vi "Radau5_Choose Step Size.vi"(0 "step size":dbl, 1 "Step index":i32, 2 "Index of Y":i8[](array[numeric]), 5 "old step size":dbl, 7 "ErrorTolerance":dbl[](array[numeric]), 9 "Local error":dbl[](array[numeric]), 11 "Old Local error":dbl[](array[numeric])) -> (4 "New step size":dbl)   [LabVIEW 2017, in "NI_DAE.lvlib"]
uses:
  <vilib>/gmath/NI_DAE.lvlib
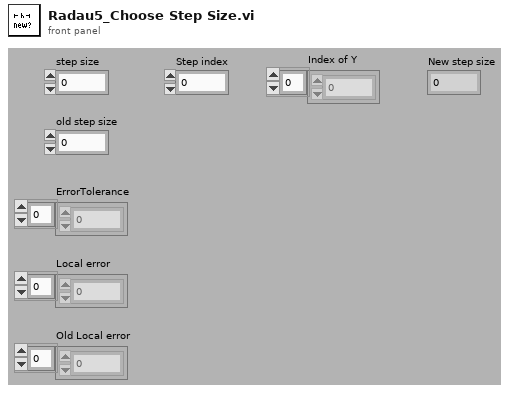
[diagram p1: front panel]
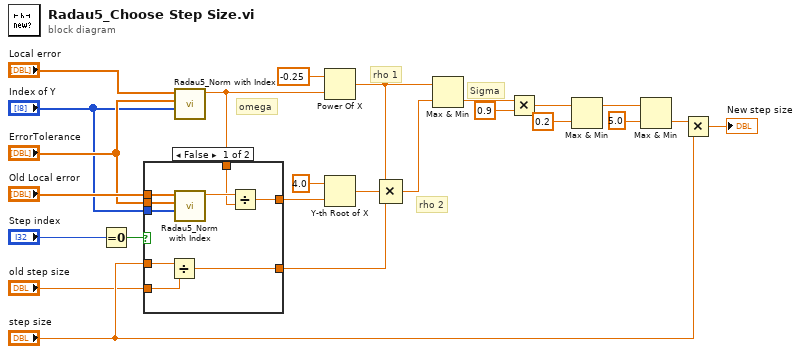
[diagram p0: block diagram]
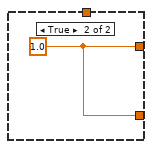
[diagram p2: hidden frame]
diagram:
  # "Sigma"
  # "rho 2"
  # "rho 1"
  # "omega"
  n1 = Equal To 0?(x="Step index") -> (x = 0?=w12:bool)
  n2 = call <vilib>:"Radau5_Norm with Index.vi"("Index of Y"="Index of Y", "ErrorTolerance"="ErrorTolerance", "Local error"="Local error") -> ("Error"=w2:dbl)  [unwired: 8 in]
  n3 = case shown="False" w12 {
    tunnel: "Old Local error" -> [w29 _]
    tunnel: [w33 w34] -> w10
    tunnel: "step size" -> [w32 _]
    tunnel: "old step size" -> [w31 _]
    tunnel: [w30 w34] -> w5
    tunnel: "ErrorTolerance" -> [w27 _]
    tunnel: w2 -> [w26 _]
    tunnel: "Index of Y" -> [w25 _]
    frame False {
      n4 = Divide(x=w32, y=w31) -> (x/y=w30:dbl)
      n5 = call <vilib>:"Radau5_Norm with Index.vi"("Index of Y"=w25, "ErrorTolerance"=w27, "Local error"=w29) -> ("Error"=w28:dbl)  [unwired: 8 in]
      n6 = Divide(x=w28, y=w26) -> (x/y=w33:dbl)
    }
    frame True {
      w34 = 1.0 ("x")
    }
  }
  n7 = Power Of X(1:w2, 2:-0.25 ("x")) -> (0:w23:dbl)
  n8 = Y-th Root of X(1:w10, 2:4.0 ("x")) -> (0:w14:dbl)
  n9 = Compound Arithmetic op=MULTIPLY(w23, w14, w5) -> (w24:dbl)
  n10 = Max & Min(x=w23, y=w24) -> (min(x,y)=w22:dbl)  [unwired: 1 out]
  n11 = Multiply(x=w22, y=0.9) -> (x*y=w20:dbl)
  n12 = Max & Min(x=w20, y=0.2) -> (max(x,y)=w18:dbl)  [unwired: 1 out]
  n13 = Max & Min(x=w18, y=5.0) -> (min(x,y)=w16:dbl)  [unwired: 1 out]
  n14 = Multiply(x=w16, y="step size") -> (x*y=→"New step size":dbl)
